vi "GetControlImageFromTabControl.vi"(8 "page":i32, 9 "control":i32, 11 "Ctl Refnum":refnum<vi>) -> (0 "error out":errorcluster, 1 "element":refnum<vi>, 3 "image data":T1)   [LabVIEW 2016]
uses:
  <vilib>/picture/picture.llb/imagedata.ctl
panel:
  in  "error in":errorcluster
  in  "TabCtl Refnum":refnum<vi>
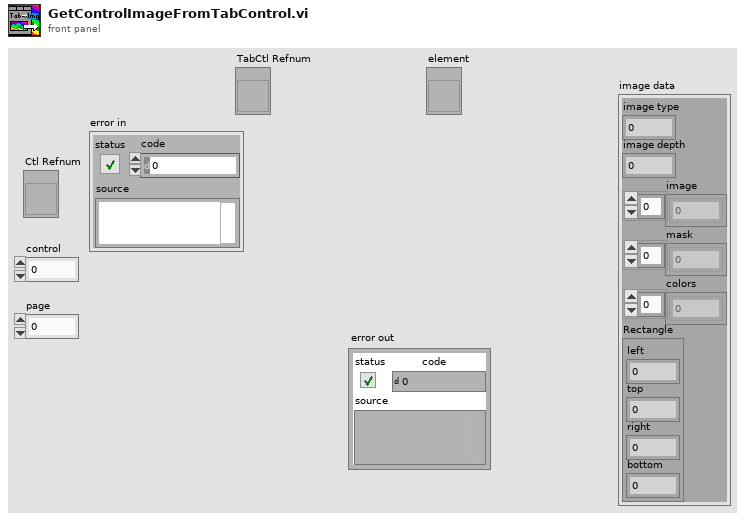
[diagram p1: front panel]
types:
  T1 = typedef "imagedata.ctl" = cluster{"image type":i32, "image depth":i32, "image":u8[], "mask":u8[], "colors":u32[], "Rectangle":cluster{"left":i16, "top":i16, "right":i16, "bottom":i16}}
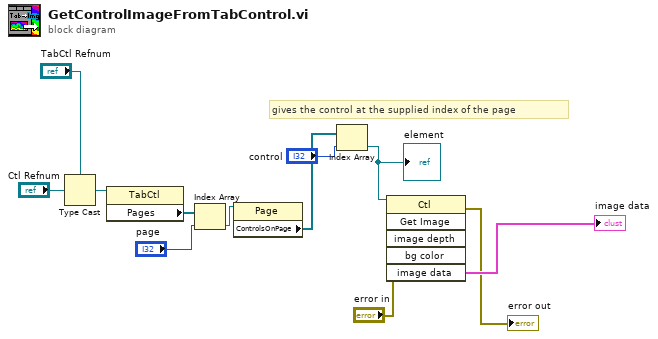
[diagram p0: block diagram]
diagram:
  # "gives the control at the supplied index of the page"
  n1 = Type Cast(type="TabCtl Refnum", x="Ctl Refnum") -> (*(type *) &x=w6:refnum<vi>)
  n2 = property class="TabCtl"(reference=w6) -> ("Pages"=w7:refnum<vi>[])  [unwired: 1 in, 2 out]
  n3 = Index Array(array=w7, index="page") -> (element=w9:refnum<vi>)
  n4 = property class="Page"(reference=w9) -> ("ControlsOnPage"=w11:refnum<vi>[])  [unwired: 1 in, 2 out]
  n5 = Index Array(array=w11, index="control") -> (element=w12:refnum<vi>)
  "element" <- w12
  n6 = invoke class="Ctl" method="Get Image"(reference=w12, error in="error in") -> (error out=→"error out":errorcluster, "image data"=→"image data":T1)  [unwired: 4 in, 4 out]
